vi "FPGAMemoryInit_SpriteIndexes_RLE_U32.vi"() -> (0 "Init Data Out":u32[](array[numeric]))   [LabVIEW 2020]
uses:
  <vilib>/Utility/file.llb/Application Directory.vi
  <vilib>/picture/bmp.llb/Read BMP File.vi
panel:
  out "RLE Images":fxp<+,12,12>[](array[numeric])
  # "For Initialization VI requirements and help, please read directions located on Block Diagram."
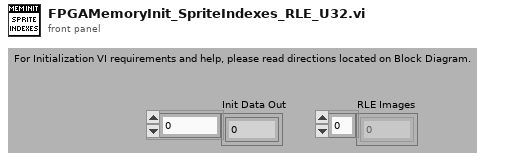
[diagram p1: front panel]
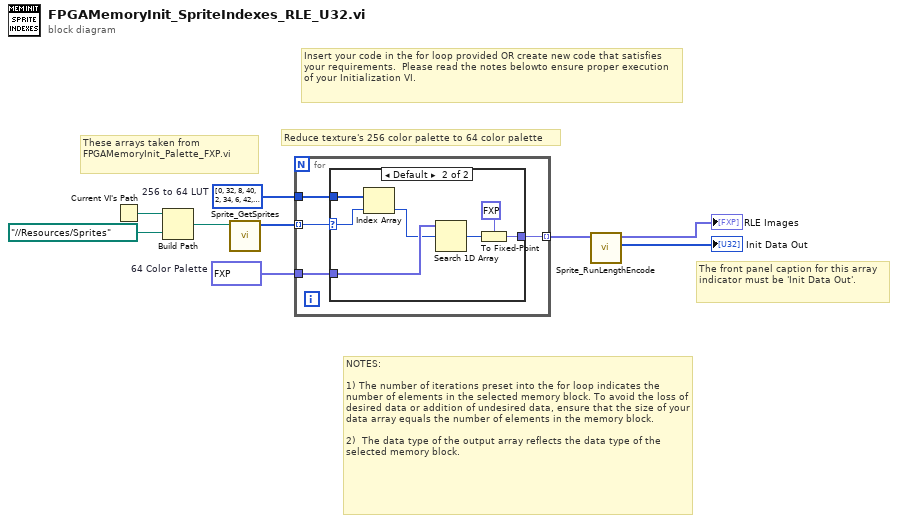
[diagram p0: block diagram]
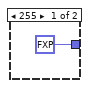
[diagram p2: hidden frame]
diagram:
  w7 = fxp<+,8,8>[] [0.0, 32.0, 8.0, 40.0, 2.0, 34.0, 6.0, 42.0, 21.0, 53.0, 29.0, 61.0, 23.0, 55.0, 31.0, 63.0, 3.0, 1.0, 43.0, 27.0, 11.0, 7.0, 47.0, 15.0, 10.0, 5.0, 30.0, 14.0, 9.0, 46.0, 12.0, 4.0, 62.0, 60.0, 20.0, 57.0, 56.0, 36.0, 58.0, 48.0, 16.0, 50.0, 33.0, 17.0, 59.0, 51.0, 26.0, 22.0, 41.0]  # 64 Color Palette
  w8 = u8[] [0, 32, 8, 40, 2, 34, 6, 42, 21, 53, 29, 61, 23, 55, 31, 63, 63, 63, 42, 42, 42, 42, 42, 42, 21, 21, 21, 21, 21, 21, 21, 0, 3, 3, 3, 2, 2, 2, 2, 2, 2, 2, 1, 1, 1, 1, 1, 1, 63, 43, 43, 23, 23, 23, 3, 3, 27, 27, 11, 7, 7, 6, 6, 6, 63, 47, 47, 31, 31, 31, 15, 15, 15, 10, 10, 10, 10, 5, 5, 5, 30, 30, 14, 14, 14, 10, 9, 9, 63, 46, 46, 30, 29, 29, 12, 12, 12, 12, 12, 8, 8, 8, 8, 8, 8, 8, 4, 4, 4, 4, 4, 4, 63, 62, 62, 61, 61, 61, 60, 60, 60, 40, 40, 40, 40, 20, 20, 20, 57, 57, 56, 56, 56, 36, 36, 36, 63, 58, 58, 57, 53, 53, 48, 48, 48, 48, 48, 32, 32, 32, 32, 32, 32, 32, 16, 16, 16, 16, 16, 16, 0, 31, 11, 11, 11, 11, 50, 50, 50, 34, 33, 33, 33, 17, 17, 16, 63, 59, 59, 55, 55, 55, 51, 51, 51, 34, 34, 34, 34, 17, 17, 17, 63, 47, 47, 43, 43, 43, 43, 43, 43, 27, 27, 27, 27, 27, 26, 22, 22, 22, 22, 22, 22, 22, 22, 22, 5, 5, 5, 5, 5, 5, 5, 0, 17, 20, 20, 0, 16, 1, 17, 17, 16, 0, 21, 21, 21, 21, 21, 63, 62, 62, 41, 41, 40, 40, 40, 40, 40, 40, 20, 20, 20, 20, 20, 34]  # 256 to 64 LUT
  # "Reduce texture's 256 color palette to 64 color palette"
  # "These arrays taken from FPGAMemoryInit_Palette_FXP.vi"
  # "The front panel caption for this array indicator must be 'Init Data Out'."
  # "NOTES:\n\n1) The number of iterations preset into the for loop indicates the number of elements in the selected memory block. To avoid the loss of desired data or addition of undesired data, ensure that the size of your data array equals the number of elements in the memory block.\n\n2)  The data type of the output array reflects the data type of the selected memory block."
  # "Insert your code in the for loop provided OR create new code that satisfies your requirements.  Please read the notes belowto ensure proper execution of your Initialization VI."
  n1 = Current VI's Path() -> (path=w6:path)
  n2 = Build Path(base path=w6, name or relative path=path "../../Resources/Sprites") -> (appended path=w4:path)
  n3 = call "Sprite_GetSprites.vi"("Sprite Path"=w4) -> ("Sprites"=w9:u8[])  [unwired: 10 in]
  n4 = for {
    tunnel: w9 -> [w10] mode=indexing
    tunnel: w8 -> [w13]
    tunnel: w7 -> [w12]
    tunnel: [w11] -> w3 mode=indexing
    n5 = case shown="Default" w10 {
      selector: w10 -> [_ w15]
      tunnel: w13 -> [_ w21]
      tunnel: w12 -> [_ w20]
      tunnel: [fxp<+,6,6> 63.0 ("fixed-point type") w17] -> w11
      frame 255 {
      }
      frame Default {
        n6 = Index Array(array=w21, index=w15) -> (element=w19:u8)
        n7 = Search 1D Array(1D array=w20, element=w19) -> (index of element=w18:i32)  [unwired: 1 in]
        n8 = To Fixed-Point(fixed-point type=fxp<+,6,6> 0.0, number=w18) -> (fixed-point=w17:fxp<+,6,6>)
      }
    }
  }
  n9 = call "Sprite_RunLengthEncode.vi"("64 Color Images (Concatenated)"=w3) -> ("Indexes"=→"Init Data Out":u32[], "RLE Images"=→"RLE Images":fxp<+,12,12>[])  [unwired: 9 in]
